vi "Target.vi"   [LabVIEW 2025]
uses:
  <vilib>/rvi/DataTransferAndStorage/Container/XNode/niFpgaContainer.xnode
  <vilib>/rvi/interface/RandomDataEmulation/nirviRandomDataFpgaReadWriteTemplate.vi
  <vilib>/rvi/Memory/Memory_Emulation/nirvimemoryEmulation.vi
  <vilib>/rvi/Memory/Memory_Emulation/nirvimemoryFastEmulation.vi
  <vilib>/rvi/DataTransferAndStorage/Register/Emulation/niFpgaRegisterEmulation.vi
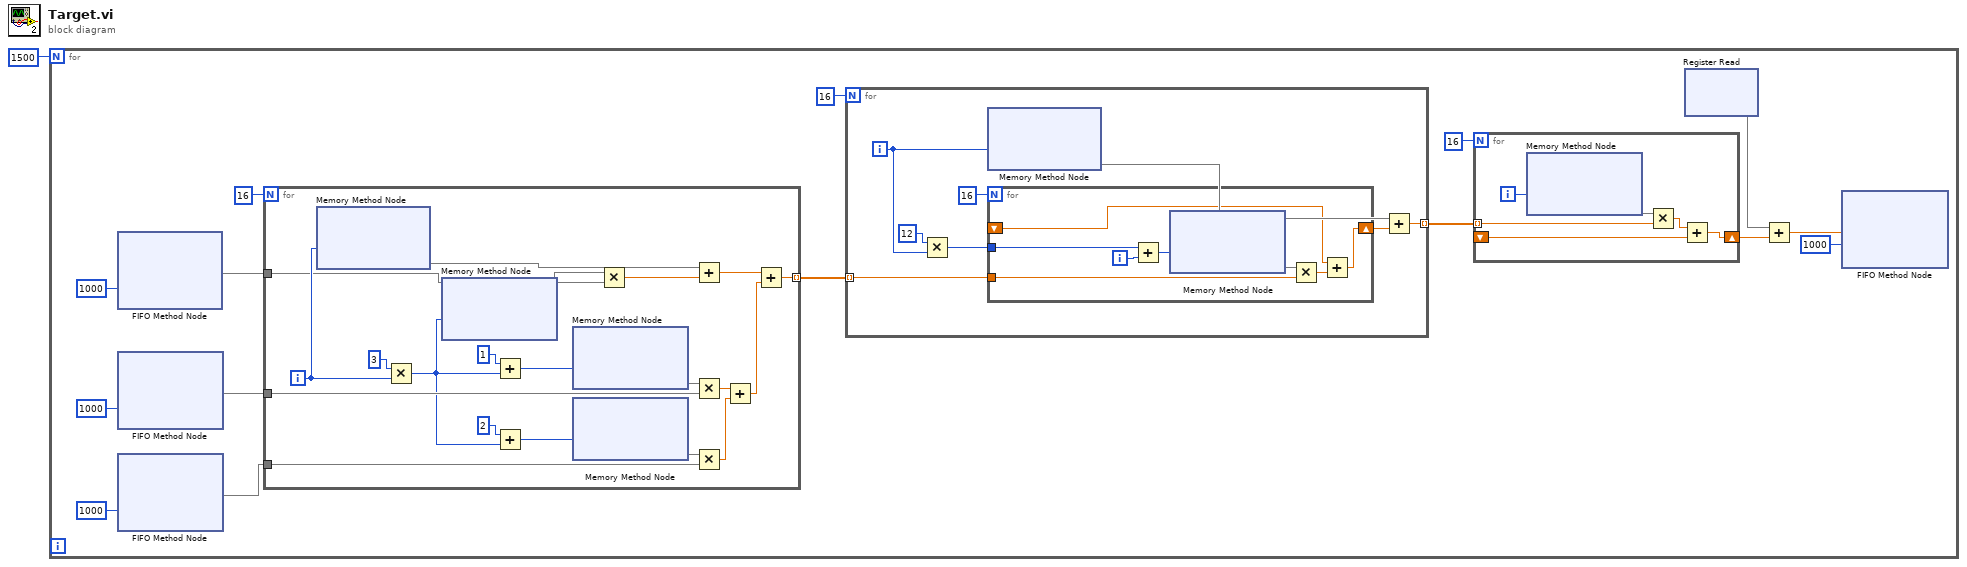
[diagram p0: block diagram]
diagram:
  n1 = for {
    N: 1500 -> [_]
    n2 = xnode ("FIFO Method Node")("Timeout"=1000) -> ("Element"=w2)  [unwired: 1 in, 2 out]
    n3 = xnode ("FIFO Method Node")("Timeout"=1000) -> ("Element"=w13)  [unwired: 1 in, 2 out]
    n4 = xnode ("FIFO Method Node")("Timeout"=1000) -> ("Element"=w12)  [unwired: 1 in, 2 out]
    n5 = for {
      N: 16 -> [_]
      tunnel: w13 -> [w58]
      tunnel: w12 -> [w57]
      tunnel: [w51] -> w10 mode=indexing
      tunnel: w2 -> [w39]
      i -> [w46]
      n6 = xnode ("Memory Method Node")("Address"=w46) -> ("Data"=w50)  [unwired: 1 in, 1 out]
      n7 = Multiply(x=3, y=w46) -> (x*y=w44:i32)
      n8 = xnode ("Memory Method Node")("Address"=w44) -> ("Data"=w49)  [unwired: 1 in, 1 out]
      n9 = Add(x=1, y=w44) -> (x+y=w40:i32)
      n10 = Add(x=2, y=w44) -> (x+y=w41:i32)
      n11 = xnode ("Memory Method Node")("Address"=w40) -> ("Data"=w48)  [unwired: 1 in, 1 out]
      n12 = xnode ("Memory Method Node")("Address"=w41) -> ("Data"=w47)  [unwired: 1 in, 1 out]
      n13 = Multiply(x=w49, y=w39) -> (x*y=w54:dbl)
      n14 = Add(x=w50, y=w54) -> (x+y=w53:dbl)
      n15 = Multiply(x=w48, y=w58) -> (x*y=w55:dbl)
      n16 = Multiply(x=w47, y=w57) -> (x*y=w56:dbl)
      n17 = Add(x=w55, y=w56) -> (x+y=w52:dbl)
      n18 = Add(x=w53, y=w52) -> (x+y=w51:dbl)
    }
    n19 = for {
      N: 16 -> [_]
      tunnel: w10 -> [w27] mode=indexing
      tunnel: [w30] -> w8 mode=indexing
      i -> [w25]
      n20 = Multiply(x=12, y=w25) -> (x*y=w26:i32)
      n21 = xnode ("Memory Method Node")("Address"=w25) -> ("Data"=w29)  [unwired: 1 in, 1 out]
      n22 = for {
        N: 16 -> [_]
        tunnel: w27 -> [w38]
        tunnel: w26 -> [w34]
        shift-right: [w32] -> w23
        shift-left: _ -> [w31]
        i -> [w36]
        n23 = Add(x=w34, y=w36) -> (x+y=w35:i32)
        n24 = xnode ("Memory Method Node")("Address"=w35) -> ("Data"=w37)  [unwired: 1 in, 1 out]
        n25 = Multiply(x=w37, y=w38) -> (x*y=w33:dbl)
        n26 = Add(x=w31, y=w33) -> (x+y=w32:dbl)
      }
      n27 = Add(x=w29, y=w23) -> (x+y=w30:dbl)
    }
    n28 = for {
      N: 16 -> [_]
      tunnel: w8 -> [w22] mode=indexing
      shift-right: [w19] -> w7
      shift-left: _ -> [w20]
      i -> [w17]
      n29 = xnode ("Memory Method Node")("Address"=w17) -> ("Data"=w18)  [unwired: 1 in, 1 out]
      n30 = Multiply(x=w18, y=w22) -> (x*y=w21:dbl)
      n31 = Add(x=w21, y=w20) -> (x+y=w19:dbl)
    }
    n32 = xnode ("Register Read")() -> ("Data"=w5)  [unwired: 1 in, 1 out]
    n33 = Add(x=w5, y=w7) -> (x+y=w6:dbl)
    n34 = xnode ("FIFO Method Node")("Element"=w6, "Timeout"=1000) -> ()  [unwired: 1 in, 2 out]
  }
